vi "Arrondir Dbl.vi"(3 "Nombre IN":dbl format="%#.10g", 4 "Décimale":u8 max=10) -> (7 "Nombre OUT":dbl format="%#.10g")   [LabVIEW 2019, in "Exaprom PDF.lvlib"]
uses:
  Exaprom PDF.lvlib
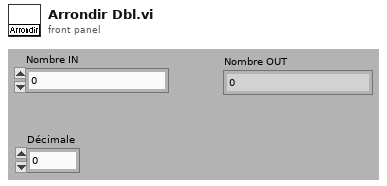
[diagram p1: front panel]
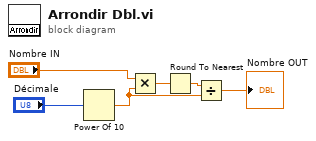
[diagram p0: block diagram]
diagram:
  n1 = Power Of 10(x="Décimale") -> (10^x=w4:dbl)
  n2 = Multiply(x="Nombre IN", y=w4) -> (x*y=w2:dbl)
  n3 = Round To Nearest(number=w2) -> (nearest integer value=w1:dbl)
  n4 = Divide(x=w1, y=w4) -> (x/y=→"Nombre OUT":dbl)
